vi "Frame2Data.vi"(10 "Frame":string) -> (0 "element":string[](array[string]), 1 "MulFrame?":bool, 2 "DataBytes":u8[](array[numeric]) format="%.0x", 3 "GetKey?":bool, 4 "Finish":bool, 5 "Error?":bool)   [LabVIEW 2018]
uses:
  <vilib>/regexp/Match Regular Expression.xnode
panel:
  out "匹配后偏移量":i32
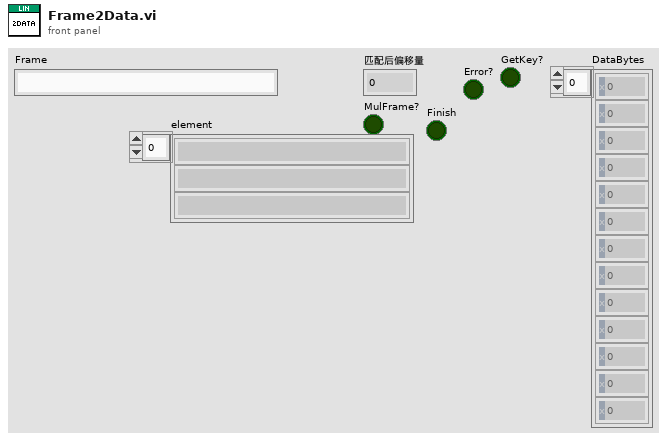
[diagram p1: front panel]
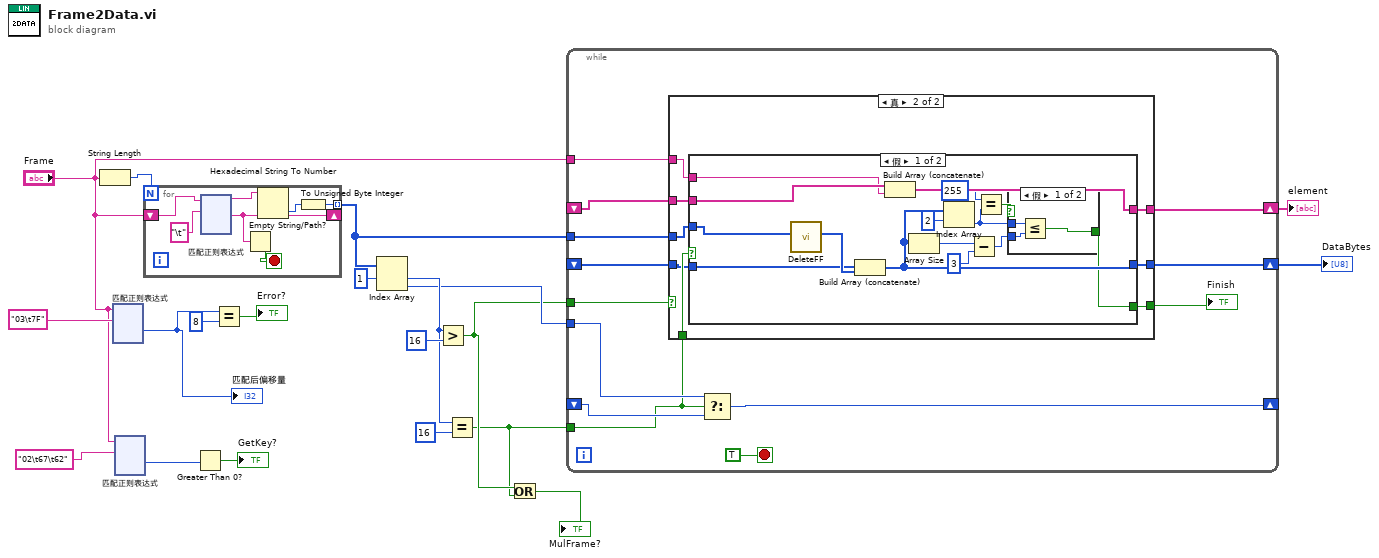
[diagram p0: block diagram]
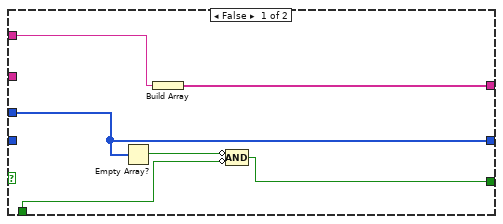
[diagram p2: hidden frame]
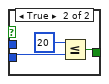
[diagram p3: hidden frame]
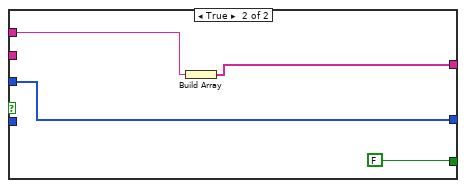
[diagram p4: hidden frame]
diagram:
  n1 = String Length(string="Frame") -> (length=w20:i32)
  n2 = xnode "匹配正则表达式"("input string"="Frame", "regular expression"="03\t7F" ("Frame")) -> ("offset past match"=w18:i32)  [unwired: 4 in, 4 out]
  "匹配后偏移量" <- w18
  n3 = xnode "匹配正则表达式"("input string"="Frame", "regular expression"="02\t67\t62" ("正则表达式")) -> ("offset past match"=w13:i32)  [unwired: 4 in, 4 out]
  n4 = for {
    N: w20 -> [_]
    shift-right: [w25] -> _
    shift-left: "Frame" -> [w27]
    tunnel: [w21] -> w7 mode=indexing
    stop <- w24 stop-if-true
    n5 = xnode "匹配正则表达式"("input string"=w27, "regular expression"="\t" ("正则表达式")) -> ("before match"=w22:string, "after match"=w25:string)  [unwired: 4 in, 3 out]
    n6 = Empty String/Path?(string/path=w25) -> (empty?=w24:bool)
    n7 = Hexadecimal String To Number(string=w22) -> (number=w23:u32)  [unwired: 2 in, 1 out]
    n8 = To Unsigned Byte Integer(number=w23) -> (unsigned 8bit integer=w21:u8)
  }
  n9 = Greater Than 0?(x=w13) -> (x > 0?=→"GetKey?":bool)
  n10 = Equal?(x=w18, y=8) -> (x = y?=→"Error?":bool)
  n11 = Index Array(array=w7, index #1=1 ("索引")) -> (element #1=w10:u8, element #2=w8:u8)  [unwired: 1 in]
  n12 = Greater?(x=w10, y=u8 16) -> (0:w3:bool)
  n13 = Equal?(x=w10, y=u8 16) -> (x = y?=w2:bool)
  n14 = Or(x=w3, y=w2) -> (x .or. y?=→"MulFrame?":bool)
  n15 = while {
    tunnel: w2 -> [w149]
    shift-right: [w153] -> _
    shift-left: _ -> [w151]
    tunnel: w8 -> [w152]
    tunnel: w3 -> [w150]
    tunnel: w7 -> [w148]
    shift-right: [w147] -> w6
    shift-left: _ -> [w146]
    tunnel: "Frame" -> [w144]
    shift-right: [w143] -> w4
    shift-left: _ -> [w142]
    stop <- TRUE stop-if-true
    n16 = case shown="真" w150 {
      tunnel: w149 -> [w155 w168]
      tunnel: w148 -> [w160 w166]
      tunnel: [w160 w167] -> w147
      tunnel: w146 -> [_ w165]
      tunnel: [w158 w164] -> w145
      tunnel: w144 -> [w157 w163]
      tunnel: [w156 w162] -> w143
      tunnel: w142 -> [_ w161]
      frame False {
        n17 = Empty Array?(array=w160) -> (empty?=w159:bool)
        n18 = Build Array(w157) -> (w156:string[])
        n19 = Compound Arithmetic op=AND ("复合运算")(invert w159, invert w155) -> (w158:bool)
      }
      frame True {
        n20 = case shown="假" w168 {
          tunnel: [w180 w193] -> w167
          tunnel: w166 -> [w169 w193]
          tunnel: w165 -> [w170 _]
          tunnel: [w177 FALSE] -> w164
          tunnel: w163 -> [w175 w191]
          tunnel: [w174 w190] -> w162
          tunnel: w161 -> [w176 _]
          frame False {
            n21 = call "DeleteFF.vi"("Data"=w169) -> ("Data out"=w183:u8[])  [unwired: 10 in]
            n22 = Build Array (concatenate)(w170, w183) -> (w180:u8[])
            n23 = Build Array (concatenate)(w176, w175) -> (w174:string[])
            n24 = Array Size(array=w180) -> (size(s)=w182:i32)
            n25 = Index Array(array=w180, index=2 ("索引")) -> (element=w173:u8)
            n26 = Subtract(x=w182, y=3) -> (x-y=w178:i32)
            n27 = Equal?(x=u8 255, y=w173) -> (x = y?=w171:bool)
            n28 = case shown="假" w171 {
              tunnel: w178 -> [w186 w188]
              tunnel: [w185 w189] -> w177
              tunnel: w173 -> [w184 _]
              frame False {
                n29 = Less Or Equal?(x=w184, y=w186) -> (x <= y?=w185:bool)
              }
              frame True {
                n30 = Less Or Equal?(x=20, y=w188) -> (x <= y?=w189:bool)
              }
            }
          }
          frame True {
            n31 = Build Array(w191) -> (w190:string[])
          }
        }
      }
    }
    "Finish" <- w145
    n32 = Select(t=w152, s=w149, f=w151) -> (s? t:f=w153:u8)
  }
  "DataBytes" <- w6
  "element" <- w4
